vi "数据录入.vi"(8 "录入字符串":string, 9 "索引":dbl, 11 "总数组":string[](array[string])) -> (2 "录入完结果的数组":string[](array[string]))   [LabVIEW 2013]
panel:
  out "数组":string[](array[string])
  in  "输入":T1
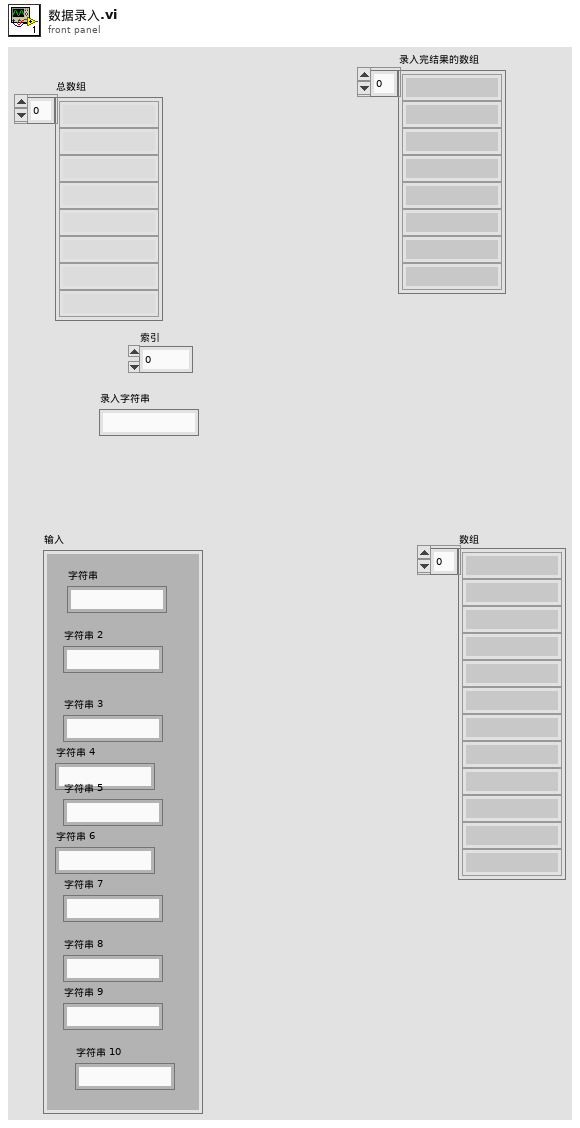
[diagram p1: front panel]
types:
  T1 = cluster{"字符串":string, "字符串 2":string, "字符串 3":string, "字符串 4":string, "字符串 5":string, "字符串 6":string, "字符串 7":string, "字符串 8":string, "字符串 9":string, "字符串 10":string}
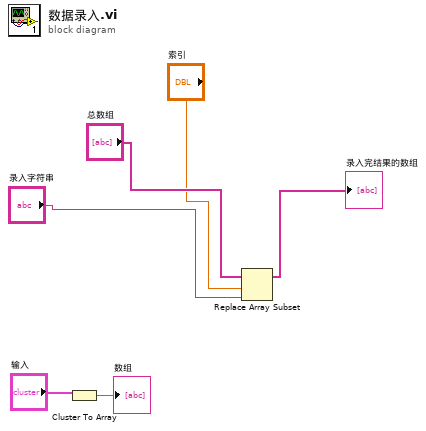
[diagram p0: block diagram]
diagram:
  n1 = Cluster To Array(cluster="输入") -> (array=→"数组":string[])
  n2 = Replace Array Subset(array="总数组", new element="录入字符串", index="索引") -> (→"录入完结果的数组":string[])
